vi "SMU Utility Function.vi"(8 "error in":errorcluster, 9 "Load Current Parameters":string[](array[string]), 10 "SMU Model":string[](array[string]), 11 "Measurement Configuration Ref":refnum<vi>) -> (0 "error out":errorcluster, 2 "Measurement Configuration Out":variant)   [LabVIEW 2021]
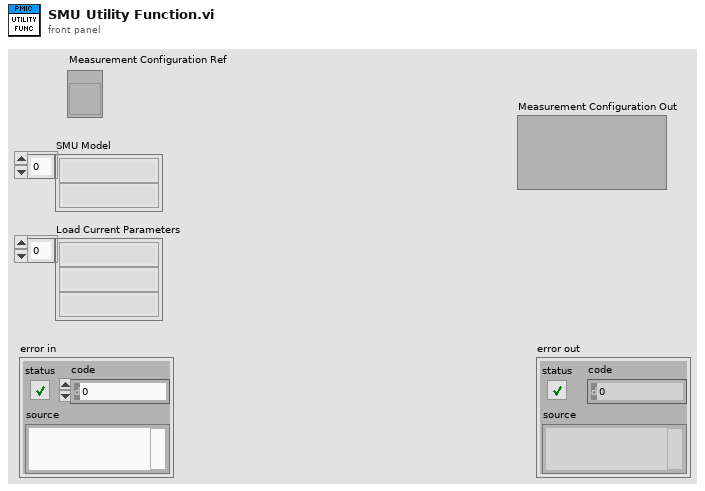
[diagram p1: front panel]
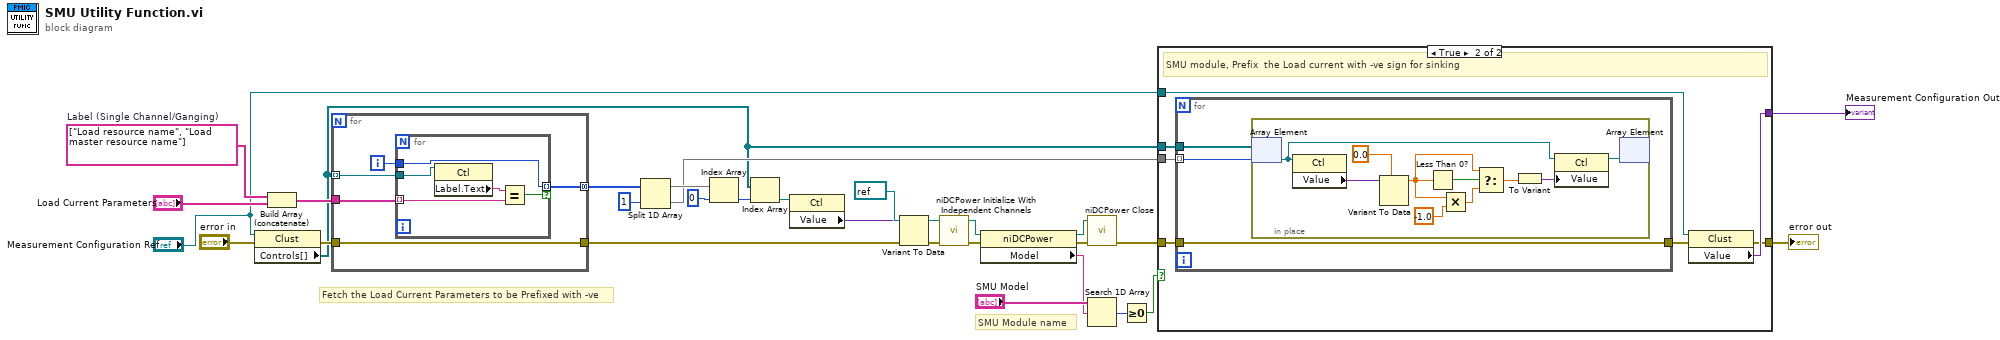
[diagram p0: block diagram]
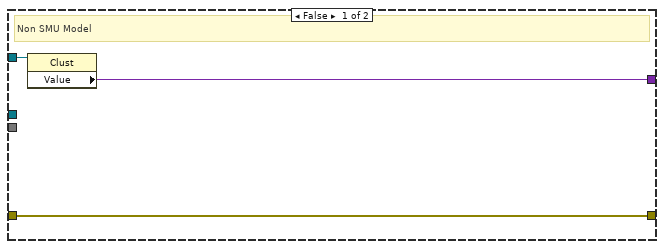
[diagram p2: hidden frame]
diagram:
  w25 = string[] ["Load resource name", "Load master resource name"]  # Label (Single Channel/Ganging)
  # "SMU Module name"
  # "Fetch the Load Current Parameters to be Prefixed with -ve"
  n1 = property class="Clust"(reference="Measurement Configuration Ref", error in="error in") -> (error out=w26:errorcluster, "Controls[]"=w15:refnum<vi>[])  [unwired: 1 out]
  n2 = Build Array (concatenate)(w25, "Load Current Parameters") -> (w24:string[])
  n3 = for {
    tunnel: w15 -> [w35] mode=indexing
    tunnel: w24 -> [w34]
    tunnel: [w32] -> w23 mode=concatenating
    tunnel: [w31] -> w13
    tunnel: w26 -> [w31]
    i -> [w33]
    n4 = for {
      tunnel: w35 -> [w40]
      tunnel: w34 -> [w38] mode=indexing
      tunnel: [w37] -> w32 mode=indexing if=w36
      tunnel: w33 -> [w37]
      n5 = property class="Ctl"(reference=w40) -> ("Label.Text"=w39:string)  [unwired: 1 in, 2 out]
      n6 = Equal?(x=w39, y=w38) -> (x = y?=w36:bool)
    }
  }
  n7 = Split 1D Array(array=w23, index=1) -> (first subarray=w21:i32[], second subarray=w16:i32[])
  n8 = Index Array(array=w21, index=0) -> (element=w19:i32)
  n9 = Index Array(array=w15, index=w19) -> (element=w18:refnum<vi>)
  n10 = property class="Ctl"(reference=w18) -> ("Value"=w1:variant)  [unwired: 1 in, 2 out]
  n11 = Variant To Data(error in=w13, type=refnum<k15> refnum ("resource name"), Variant=w1) -> (data=w10:refnum<k15>, error out=w4:errorcluster)
  n12 = call <instrlib>:"niDCPower Initialize With Independent Channels.vi"("error in (no error)"=w4, "resource name"=w10) -> ("error out"=w3:errorcluster, "instrument handle out"=w9:refnum<k15>)  [unwired: 8 in]
  n13 = property class="niDCPower"(reference=w9, error in=w3) -> (reference out=w5:refnum<k15>, error out=w2:errorcluster, "Model"=w7:string)
  n14 = call <instrlib>:"niDCPower Close.vi"("error in (no error)"=w2, "instrument handle"=w5) -> ("error out"=w29:errorcluster)  [unwired: 9 in]
  n15 = Search 1D Array(1D array="SMU Model", element=w7) -> (index of element=w6:i32)  [unwired: 1 in]
  n16 = Greater Or Equal To 0?(x=w6) -> (x >= 0?=w30:bool)
  n17 = case shown="True" w30 {
    tunnel: [w41 w50] -> w14
    tunnel: w29 -> [w43 w49]
    tunnel: [w43 w47] -> w28
    tunnel: w16 -> [_ w45]
    tunnel: w15 -> [_ w46]
    tunnel: "Measurement Configuration Ref" -> [w42 w44]
    frame False {
      # "Non SMU Model"
      n18 = property class="Clust"(reference=w42) -> ("Value"=w41:variant)  [unwired: 1 in, 2 out]
    }
    frame True {
      # "SMU module, Prefix  the Load current with -ve sign for sinking"
      n19 = for {
        tunnel: w46 -> [w53]
        tunnel: w45 -> [w52] mode=indexing
        tunnel: w49 -> [w51]
        tunnel: [w51] -> w48
        n20 = in-place {
          n21 = in-place-array #1(w53, w52) -> (w56:refnum<vi>)
          n22 = property class="Ctl"(reference=w56) -> ("Value"=w63:variant)  [unwired: 1 in, 2 out]
          n23 = Variant To Data(type=0.0, Variant=w63) -> (data=w59:dbl)  [unwired: 1 in, 1 out]
          n24 = Less Than 0?(x=w59) -> (x < 0?=w60:bool)
          n25 = Multiply(x=w59, y=-1.0) -> (x*y=w58:dbl)
          n26 = Select(t=w59, s=w60, f=w58) -> (s? t:f=w57:dbl)
          n27 = To Variant(anything=w57) -> (Variant=w55:variant)
          n28 = property class="Ctl"(reference=w56, "Value"=w55) -> (reference out=w54:refnum<vi>)  [unwired: 1 in, 1 out]
          n29 = in-place-array #1(w54) -> ()  [unwired: 2 out]
        }
      }
      n30 = property class="Clust"(reference=w44, error in=w48) -> (error out=w47:errorcluster, "Value"=w50:variant)  [unwired: 1 out]
    }
  }
  "error out" <- w28
  "Measurement Configuration Out" <- w14
